vi "Configure Probe.vi"(8 "error in (no error)":errorcluster, 10 "Tool Operation Config":T1={"Use Tool Cfg"=FALSE, "Use Tool Cal"=FALSE, "Fake Data?"=FALSE, "Mode"=-2, "Array Subset Length"=30, "nArrays to Read"=2, "Full Array Read Length"=500, "nSubarrays/Sensor"=0}) -> (0 "error out":errorcluster, 2 "Tool Operation Config out":T1={"Use Tool Cfg"=FALSE, "Use Tool Cal"=FALSE, "Fake Data?"=FALSE, "Mode"=-2, "Array Subset Length"=30, "nArrays to Read"=2, "Full Array Read Length"=500, "nSubarrays/Sensor"=0})   [LabVIEW 2015, in "Tool Module.lvlib"]
uses:
  Tool Module.lvlib
  Tool Config/_Tool Operation Config Cluster--typedef.ctl
  Tool Config/Tool Cfg.lvlib
  Tool Interface/Tool Interface.lvlib
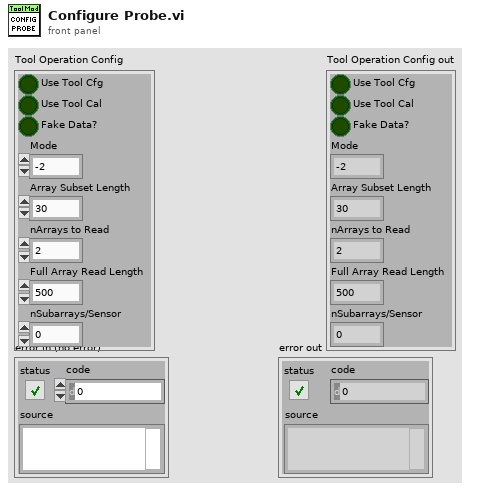
[diagram p1: front panel]
types:
  T1 = typedef "Tool Cfg.lvlib/_Tool Operation Config Cluster--typedef.ctl" = cluster{"Use Tool Cfg":bool, "Use Tool Cal":bool, "Fake Data?":bool, "Mode":i16, "Array Subset Length":i16, "nArrays to Read":i16, "Full Array Read Length":i16, "nSubarrays/Sensor":i16}
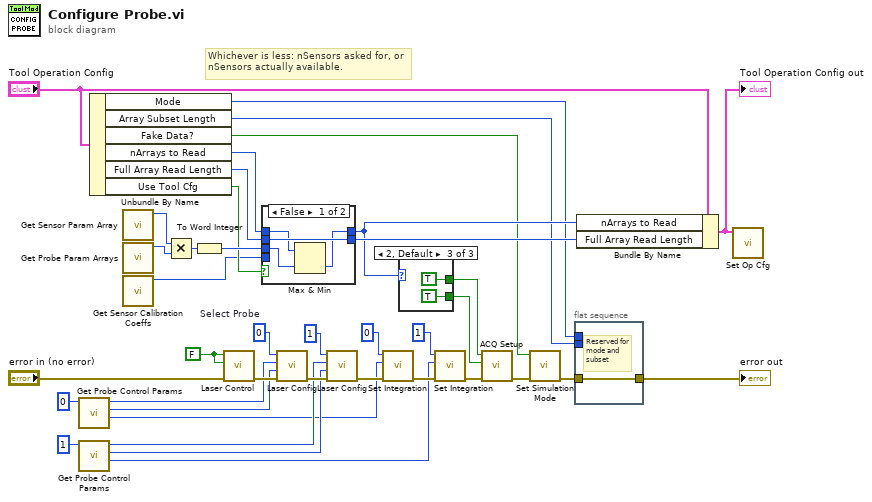
[diagram p0: block diagram]
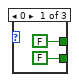
[diagram p2: hidden frame]
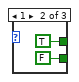
[diagram p3: hidden frame]
diagram:
  w24 = 0  # Select Probe
  w25 = FALSE ("Laser 1")
  # "Whichever is less: nSensors asked for, or nSensors actually available."
  n1 = call "Get Probe Control Params.vi"("Probe Select"=0) -> ("Integ Count"=w9:u16, "Laser Gain"=w22:u8, "Laser Init Pwr"=w23:u16)  [unwired: 8 in]
  n2 = call "Get Probe Control Params.vi"("Probe Select"=1) -> ("Integ Count"=w8:u16, "Laser Gain"=w18:u8, "Laser Init Pwr"=w19:u16)  [unwired: 8 in]
  n3 = Unbundle By Name("Tool Operation Config") -> ("Mode"=w3:i16, "Array Subset Length"=w4:i16, "Fake Data?"=w6:bool, "nArrays to Read"=w39:i16, "Full Array Read Length"=w38:i16, "Use Tool Cfg"=w33:bool)
  n4 = call "Get Sensor Param Array.vi"() -> ("Sensor Block.nSensors"=w32:u16)  [unwired: 10 in, 1 out]
  n5 = call "Get Probe Param Arrays.vi"() -> ("Probe Block.nProbes"=w31:u16)  [unwired: 10 in, 1 out]
  n6 = call "Get Sensor Calibration Coeffs.vi"() -> ("Total Pixels"=w30:u16)  [unwired: 10 in, 1 out]
  n7 = Multiply(x=w32, y=w31) -> (x*y=w37:u16)
  n8 = To Word Integer(number=w37) -> (16bit integer=w36:i16)
  n9 = call "Laser Control.vi"("error in (no error)"="error in (no error)", "Laser 2"=w25, "Laser 1"=w25) -> ("error out"=w27:errorcluster)  [unwired: 8 in]
  n10 = case shown="False" w33 {
    tunnel: [w40 w45] -> w17
    tunnel: [w43 w44] -> w34
    tunnel: w39 -> [w42 _]
    tunnel: w38 -> [w43 _]
    tunnel: w36 -> [w41 w45]
    tunnel: w30 -> [_ w44]
    frame False {
      n11 = Max & Min(x=w42, y=w41) -> (min(x,y)=w40:i16)  [unwired: 1 out]
    }
    frame True {
    }
  }
  n12 = call "Laser Config.vi"("error in (no error)"=w27, "Gain"=w22, "Init Power"=w23, "Select Probe"=w24) -> ("error out"=w21:errorcluster)  [unwired: 7 in]
  n13 = call "Laser Config.vi"("error in (no error)"=w21, "Gain"=w18, "Init Power"=w19, "Select Probe"=1) -> ("error out"=w11:errorcluster)  [unwired: 7 in]
  n14 = call "Set Integration.vi"("error in (no error)"=w11, "Integ Count"=w9, "Mode"=0 ("Select Probe")) -> ("error out"=w13:errorcluster)  [unwired: 8 in]
  n15 = case shown="2, Default" w17 {
    tunnel: [FALSE TRUE TRUE] -> w16
    tunnel: [FALSE FALSE TRUE] -> w15
    frame 0 {
    }
    frame 1 {
    }
    frame 2, Default {
    }
  }
  n16 = call "Set Integration.vi"("error in (no error)"=w13, "Integ Count"=w8, "Mode"=1 ("Select Probe")) -> ("error out"=w10:errorcluster)  [unwired: 8 in]
  n17 = call "ACQ Setup.vi"("error in (no error)"=w10, "Sensor 2"=w15, "Sensor 1"=w16) -> ("error out"=w7:errorcluster)  [unwired: 8 in]
  n18 = call "Set Simulation Mode.vi"("error in (no error)"=w7, "Simulate On"=w6) -> ("error out"=w5:errorcluster)  [unwired: 9 in]
  n19 = flat-sequence {
    tunnel: w5 -> [w52]
    tunnel: [w52] -> w2
    tunnel: w4 -> [_]
    tunnel: w3 -> [_]
    frame #0 {
      # "Reserved for mode and subset"
    }
  }
  n20 = Bundle By Name(cluster="Tool Operation Config", "nArrays to Read"=w17, "Full Array Read Length"=w34) -> (w1:T1)
  "Tool Operation Config out" <- w1
  n21 = call "Set Op Cfg.vi"("Tool Operation Config"=w1) -> ()  [unwired: 11 in]
  "error out" <- w2
